vi "Analyze Event Step 1 (40MHz).vi"(7 "measure settings.<user name>":T4, 8 "register bus":T2={"Speed"="Speed", "Crank Angle"="Crank Angle", "Cycle Angle"="Cycle Angle", "Crank Count"="Crank Count", "Cycle Count"="Cycle Count", "1.25 MHz Counter"="1.25 MHz Counter", "Crank Rollover"="Crank Rollover", "Cycle Rollover"="Cycle Rollover", "shared settings"={"start"=0.0, "stuck limit"=0.0}} {"shared settings"."start" format="%#.15g"}, 10 "event":bool) -> (3 "windowed event data":T1)   [LabVIEW 2015, in "Engine Simulation Toolkit.lvlib" / "ECU Event Timing.lvlib"]
uses:
  ECU Event Timing.lvlib
  Measure Settings.ctl
  APU/Register Bus.ctl
  APU/Shared Settings.ctl
  Windowed Event Data.ctl
  <vilib>/Utility/error.llb/Clear Errors.vi
  <vilib>/rvi/Emulation/niFpgaSctlEmulationGetInTimedLoop.vi
  <vilib>/rvi/DataTransferAndStorage/Container/Common/niFpgaContainerExecOnDevCompGetState.vi
  <vilib>/rvi/Emulation/niFpgaEmulationIsFPGAContextNoSignature.vi
  <vilib>/rvi/DataTransferAndStorage/Container/Common/niFpgaContainerGetUniqueNameForEmu.vi
  <vilib>/rvi/Memory/Memory_Emulation/niFpgaMemoryEmulationCacheClearOnFirstRun.vi
  <vilib>/rvi/Memory/Memory_Emulation/nirvimemoryEmulationManagerCache_MakeExclusive.vi
  <vilib>/rvi/Memory/Memory_Emulation/niFpgaMemoryEmulationValidateCache.vi
  <vilib>/rvi/Memory/Memory_Emulation/nirvimemoryEmulationManagerCache_InsertValue.vi
  <vilib>/rvi/Memory/Memory_Emulation/nirvimemoryEmulationManagerCache_ReleaseExclusive.vi
  <vilib>/rvi/Memory/Memory_Emulation/nirvimemoryEmulationManagerCache_GetValue.vi
  <vilib>/rvi/Memory/Memory_Emulation/nirvimemoryEmulationManagerCache_SetValue.vi
  <vilib>/rvi/Emulation/niFpgaProcessEmulError.vi
  <vilib>/rvi/DataTransferAndStorage/Container/XNode/niFpgaContainer.xnode
  <vilib>/rvi/DataTransferAndStorage/Register/Emulation/niFpgaRegisterEmulationRefIn.vi
  Engine Simulation Toolkit.lvlib
  APU/APU.lvlib
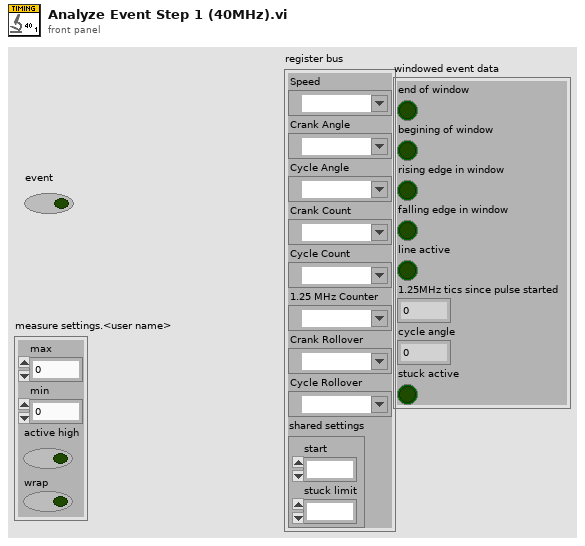
[diagram p1: front panel]
types:
  T1 = typedef "Engine Simulation Toolkit.lvlib/ECU Event Timing.lvlib/Windowed Event Data.ctl" = cluster{"end of window":bool, "begining of window":bool, "rising edge in window":bool, "falling edge in window":bool, "line active":bool, "1.25MHz tics since pulse started":fxp<+,18,18>, "cycle angle":u16, "stuck active":bool}
  T2 = typedef "Engine Simulation Toolkit.lvlib/APU.lvlib/Register Bus.ctl" = cluster{"Speed":refnum<k21>, "Crank Angle":refnum<k21>, "Cycle Angle":refnum<k21>, "Crank Count":refnum<k21>, "Cycle Count":refnum<k21>, "1.25 MHz Counter":refnum<k21>, "Crank Rollover":refnum<k21>, "Cycle Rollover":refnum<k21>, "shared settings":T3}
  T3 = typedef "Engine Simulation Toolkit.lvlib/APU.lvlib/Shared Settings.ctl" = cluster{"start":fxp<+,17,17>, "stuck limit":fxp<+,18,18>}
  T4 = typedef "Engine Simulation Toolkit.lvlib/ECU Event Timing.lvlib/Measure Settings.ctl" = cluster{"max":u16, "min":u16, "active high":bool, "wrap":bool}
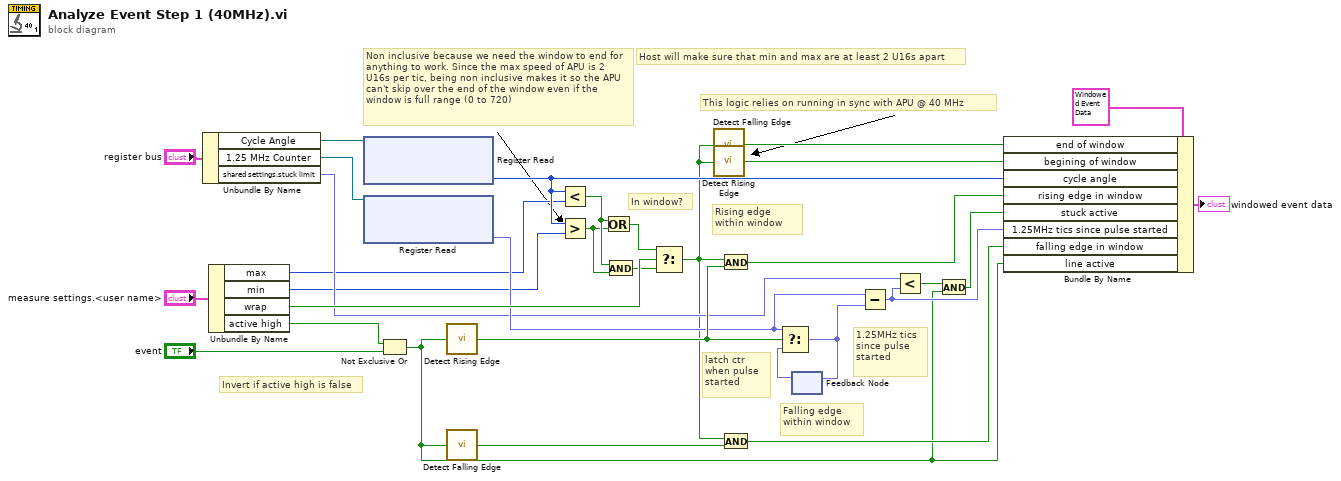
[diagram p0: block diagram]
diagram:
  # "Host will make sure that min and max are at least 2 U16s apart"
  # "Non inclusive because we need the window to end for anything to work. Since the max speed of APU is 2 U16s per tic, being non inclusive makes it so the APU can't skip over the end of the window even if the window is full range (0 to 720)"
  # "This logic relies on running in sync with APU @ 40 MHz"
  # "latch ctr when pulse started"
  # "1.25MHz tics since pulse started"
  # "Falling edge within window"
  # "Rising edge within window"
  # "Invert if active high is false"
  # "In window?"
  n1 = Unbundle By Name("register bus") -> ("Cycle Angle"=w29:refnum<k21>, "1.25 MHz Counter"=w20:refnum<k21>, "shared settings.stuck limit"=w7:fxp<+,18,18>)
  n2 = Unbundle By Name("measure settings.<user name>") -> ("max"=w5:u16, "min"=w4:u16, "wrap"=w23:bool, "active high"=w26:bool)
  n3 = xnode ("Register Read")("Register In"=w29) -> ("Data"=w6:u16)  [unwired: 1 out]
  n4 = xnode ("Register Read")("Register In"=w20) -> ("Data"=w17:fxp<+,18,18>)  [unwired: 1 out]
  n5 = Not Exclusive Or(1:"event", 2:w26) -> (0:w8:bool)
  n6 = call "Detect Rising Edge.vi"("signal"=w8) -> ("edge detected"=w19:bool)  [unwired: 14 in]
  n7 = call "Detect Falling Edge.vi"("signal"=w8) -> ("edge detected"=w27:bool)  [unwired: 14 in]
  n8 = Less?(x=w6, y=w5) -> (x < y?=w25:bool)
  n9 = Greater?(x=w6, y=w4) -> (0:w24:bool)
  n10 = Or(x=w25, y=w24) -> (x .or. y?=w22:bool)
  n11 = And(x=w25, y=w24) -> (x .and. y?=w21:bool)
  n12 = Select(t=w22, s=w23, f=w21) -> (s? t:f=w2:bool)
  n13 = call "Detect Falling Edge.vi"("signal"=w2) -> ("edge detected"=w1:bool)  [unwired: 14 in]
  n14 = call "Detect Rising Edge.vi"("signal"=w2) -> ("edge detected"=w3:bool)  [unwired: 14 in]
  n15 = And(x=w2, y=w19) -> (x .and. y?=w14:bool)
  n16 = And(x=w2, y=w27) -> (x .and. y?=w13:bool)
  n17 = feedback #1() -> (w18:fxp<+,18,18>)  [unwired: 1 in]
  n18 = Select(t=w17, s=w19, f=w18) -> (s? t:f=w16:fxp<+,18,18>)
  n19 = feedback-in #1(w16) -> ()
  n20 = Subtract(x=w17, y=w16) -> (x-y=w11:fxp<+,18,18>)
  n21 = Less?(x=w7, y=w11) -> (x < y?=w10:bool)
  n22 = And(x=w10, y=w8) -> (x .and. y?=w9:bool)
  n23 = Bundle By Name(cluster=T1 {"end of window"=FALSE, "begining of window"=FALSE, "rising edge in window"=FALSE, "falling edge in window"=FALSE, "line active"=FALSE, "1.25MHz tics since pulse started"=0.0, "cycle angle"=0, "stuck active"=FALSE} ("Windowed event data"), "end of window"=w1, "begining of window"=w3, "cycle angle"=w6, "rising edge in window"=w14, "stuck active"=w9, "1.25MHz tics since pulse started"=w11, "falling edge in window"=w13, "line active"=w8) -> (→"windowed event data":T1)
